vi "Operational.vi"(8 "error in (no error)":errorcluster, 11 "Acquisition in":refnum<class "Acquisition.lvclass">) -> (0 "error out":errorcluster, 3 "Acquisition out":refnum<class "Acquisition.lvclass">)   [LabVIEW 2018, in "Acquisition.lvclass"]
uses:
  Acquisition.lvclass
  Acquisition.lvclass/Acquisition.ctl
  Server/Server.lvclass
  Channel/Channel.lvclass
  Interface/Interface.lvclass
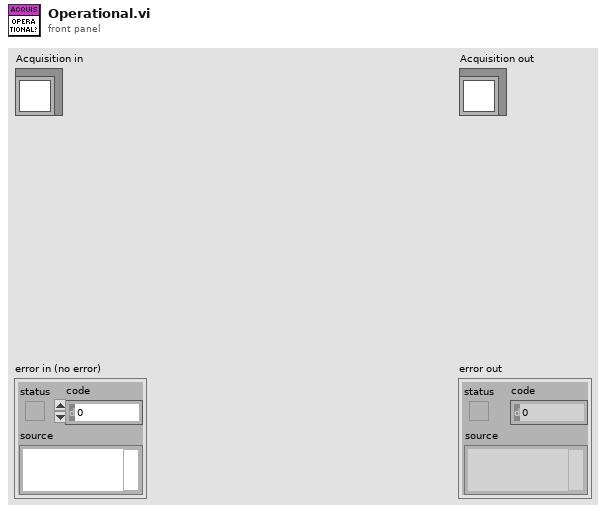
[diagram p1: front panel]
types:
  T1 = cluster{"Texp":dbl, "Nimages":u32, "InitialLine":u32, "FinalLine":u32, "InitialColumn":u32, "FinalColumn":u32, "EmGain":u32, "Cooler Off":bool, "CyclesDone":u32, "SequesDone":u32, "UsedDiskSpace":u16, "Error":bool}
  T2 = cluster{"S4GUI":bool, "S4ICS":bool, "TCS":bool, "Weather Station":bool, "Tel. focuser":bool}
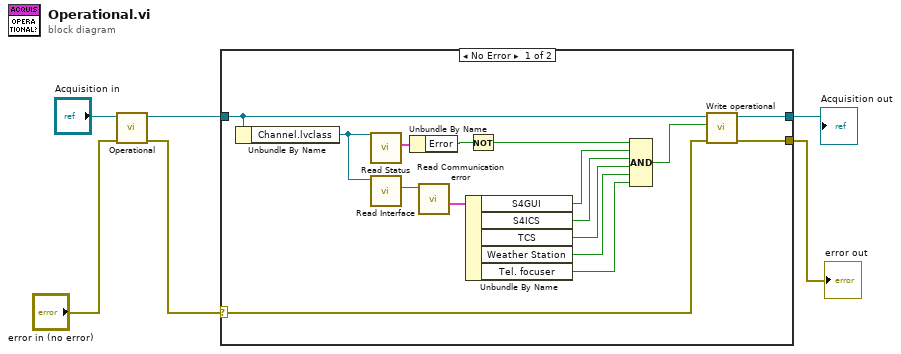
[diagram p0: block diagram]
diagram:
  n1 = call-parent "Operational.vi"("error in (no error)"="error in (no error)", "Server in"="Acquisition in") -> ("error out"=w4:errorcluster, "Server out"=w3:refnum<class "Acquisition.lvclass">)  [unwired: 8 in]
  n2 = case shown="No Error" w4 {
    selector: w4 -> [w19 w23]
    tunnel: w3 -> [w22 w24]
    tunnel: [w18 w23] -> w2
    tunnel: [w17 w24] -> w1
    frame No Error {
      n3 = Unbundle By Name(w22) -> ("Channel.lvclass"=w14:refnum<class "Channel.lvclass">)
      n4 = call-dynamic "Read Status.vi"("Channel in"=w14) -> ("Status"=w21:T1)  [unwired: 8 in, 2 out]
      n5 = call-dynamic "Read Interface.vi"("Channel in"=w14) -> ("Interface.lvclass"=w13:refnum<class "Interface.lvclass">)  [unwired: 8 in, 2 out]
      n6 = Unbundle By Name(w21) -> ("Error"=w20:bool)
      n7 = call-dynamic "Read Communication error.vi"("Interface in"=w13) -> ("Communication error"=w12:T2)  [unwired: 8 in, 2 out]
      n8 = Unbundle By Name(w12) -> ("S4GUI"=w11:bool, "S4ICS"=w10:bool, "TCS"=w7:bool, "Weather Station"=w9:bool, "Tel. focuser"=w8:bool)
      n9 = Not(x=w20) -> (.not. x?=w16:bool)
      n10 = Compound Arithmetic op=AND(w16, w11, w10, w7, w9, w8) -> (w15:bool)
      n11 = call-dynamic "Write operational.vi"("error in (no error)"=w19, "operational"=w15, "Server in"=w22) -> ("error out"=w18:errorcluster, "Server out"=w17:refnum<class "Acquisition.lvclass">)  [unwired: 7 in]
    }
    frame Error {
    }
  }
  "error out" <- w2
  "Acquisition out" <- w1
